vi "frontPanel.vi"(8 "error in (no error)":errorcluster, 10 "ScriptEvent":refnum<class "ScriptEvent.lvclass">, 11 "ActionPanel in":refnum<class "SingleToneRampAction.lvclass">) -> (0 "error out":errorcluster, 2 "ScriptEvent out":refnum<class "ScriptEvent.lvclass">, 3 "SingleToneRampAction out":refnum<class "SingleToneRampAction.lvclass">)   [LabVIEW 2011, in "Views.lvlib" / "ScriptEditor.lvlib" / "SingleToneRampAction.lvclass"]
uses:
  SingleToneRampAction.lvclass
  Tools/Scripting/ScriptingEvent/ScriptEvent.lvclass
  SingleToneRampAction.lvclass/SingleToneRampAction.ctl
  Tools/Scripting/ScriptingEvent/ScriptEvents/SingleTone/SingleToneRamp/SingleToneRamp.lvclass
  ActionPanel.lvclass
  Tools/Scripting/ScriptingEvent/ScriptEvents/SingleTone/SingleTone.lvclass
panel:
  in  "Stop Phase (Degrees)":dbl format="%#.6g"
  in  "Stop Frequency (kHz)":dbl format="%#.6g"
  in  "Stop Amplitude (Vpp)":string
  in  "Ramp Time":dbl format="%.6g"
  in  "Start Phase (Degrees)":dbl format="%#.6g"
  in  "Start Frequency (kHz)":dbl format="%#.6g"
  in  "Time":dbl format="%.6g"
  in  "Start Amplitude (Vpp)":string
  in  "Dt":dbl format="%.6g"
  out "editing":bool
  out "ready?":bool
  in  "close":bool
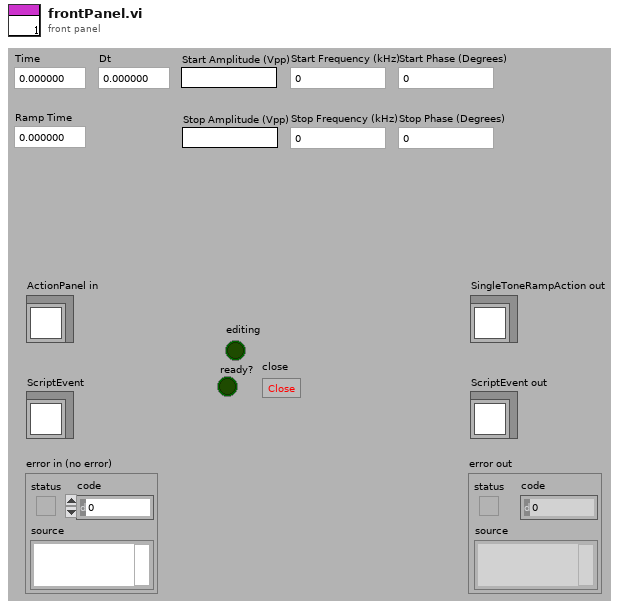
[diagram p1: front panel]
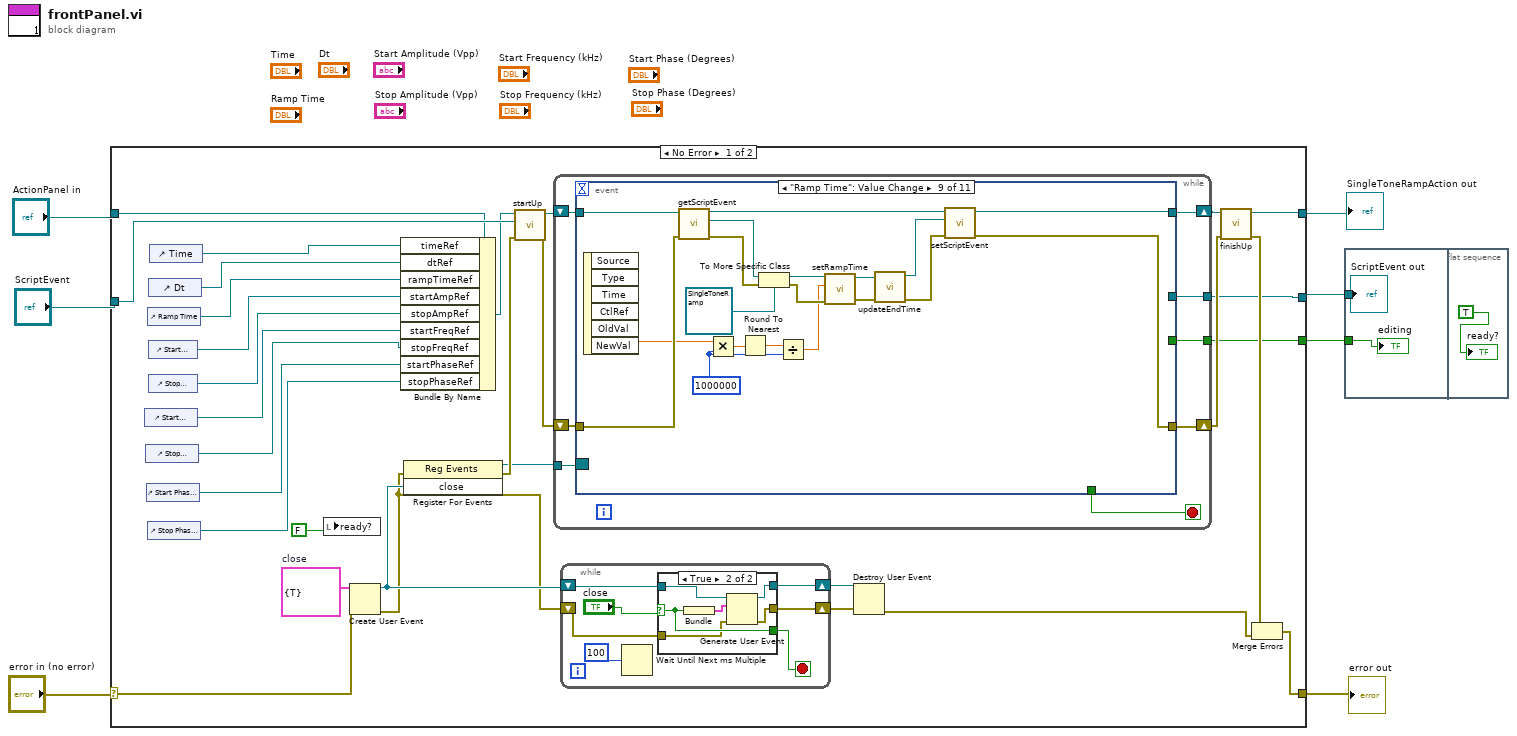
[diagram p0: block diagram]
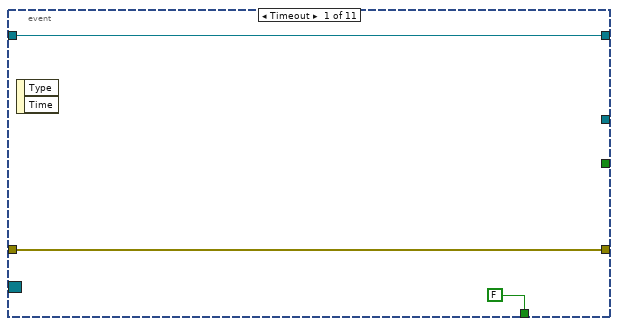
[diagram p3: hidden frame]
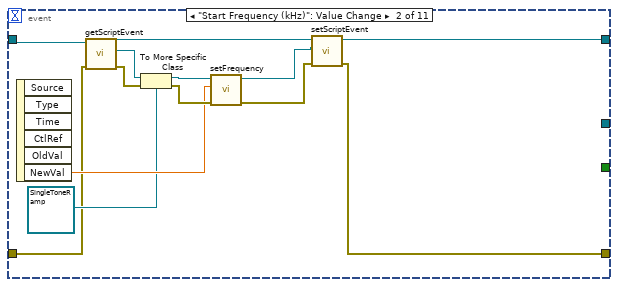
[diagram p4: hidden frame]
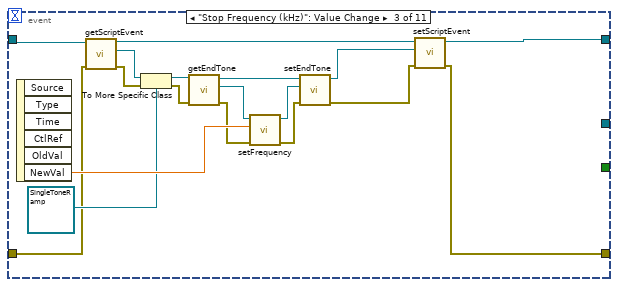
[diagram p5: hidden frame]
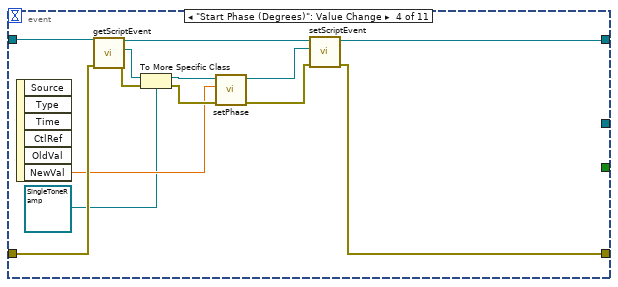
[diagram p6: hidden frame]
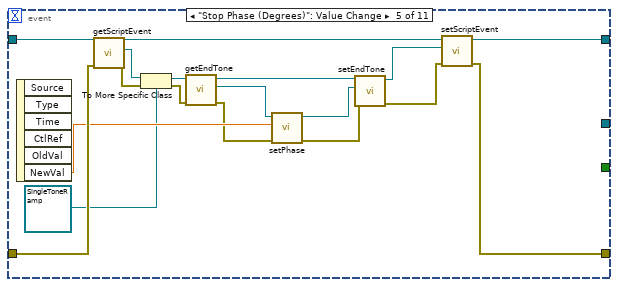
[diagram p7: hidden frame]
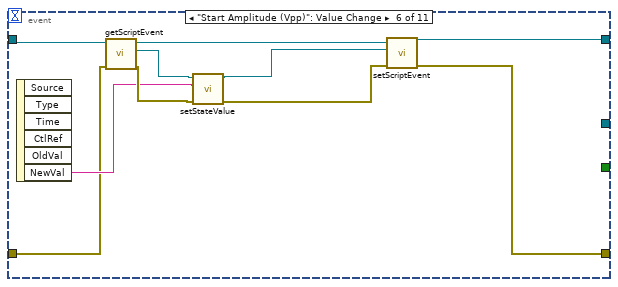
[diagram p8: hidden frame]
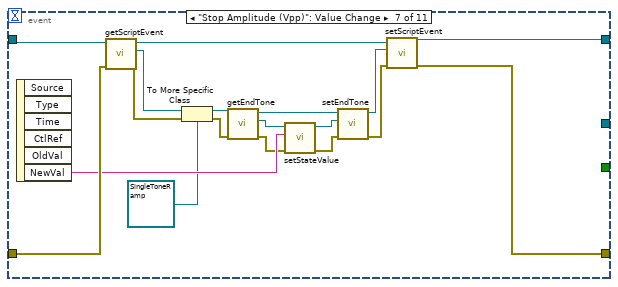
[diagram p9: hidden frame]
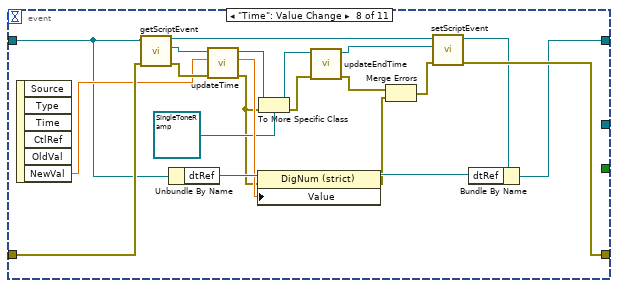
[diagram p10: hidden frame]
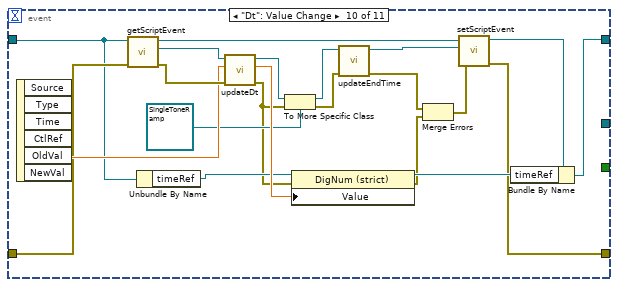
[diagram p11: hidden frame]
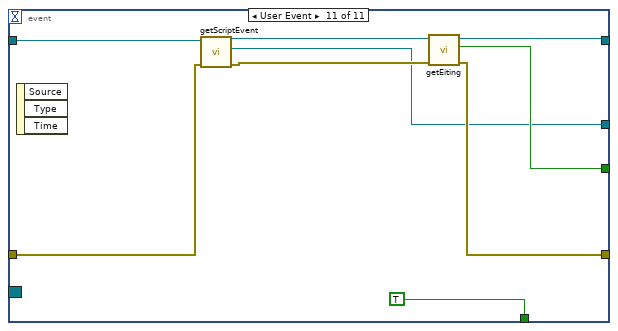
[diagram p12: hidden frame]
diagram:
  n1 = case shown="No Error" "error in (no error)" {
    selector: "error in (no error)" -> [w26 w226]
    tunnel: [w28 w226] -> w6
    tunnel: "ActionPanel in" -> [w9 w228]
    tunnel: [w38 w228] -> w1
    tunnel: "ScriptEvent" -> [w33 w227]
    tunnel: [w21 w227] -> w7
    tunnel: [w20 _] -> w2
    frame No Error {
      w27 = cluster{"close":bool} {"close"=TRUE}  # close
      n2 = control-ref of="Start Frequency (kHz)"() -> (w13:refnum<vi>)
      n3 = control-ref of="Stop Frequency (kHz)"() -> (w12:refnum<vi>)
      n4 = control-ref of="Start Phase (Degrees)"() -> (w11:refnum<vi>)
      n5 = control-ref of="Ramp Time"() -> (w16:refnum<vi>)
      n6 = control-ref of="Stop Phase (Degrees)"() -> (w10:refnum<vi>)
      n7 = control-ref of="Dt"() -> (w18:refnum<vi>)
      n8 = control-ref of="Start Amplitude (Vpp)"() -> (w15:refnum<vi>)
      n9 = control-ref of="Stop Amplitude (Vpp)"() -> (w14:refnum<vi>)
      n10 = control-ref of="Time"() -> (w19:refnum<vi>)
      n11 = local write "ready?"(FALSE) -> ()
      n12 = Create User Event(user event datatype=w27, error in=w26) -> (user event=w25:refnum<user-event>, error out=w24:errorcluster)
      n13 = Bundle By Name(cluster=w9, "timeRef"=w19, "dtRef"=w18, "rampTimeRef"=w16, "startAmpRef"=w15, "stopAmpRef"=w14, "startFreqRef"=w13, "stopFreqRef"=w12, "startPhaseRef"=w11, "stopPhaseRef"=w10) -> (w8:refnum<class "SingleToneRampAction.lvclass">)
      n14 = register-events(error in=w24, w25) -> (reference out=w22:refnum<event-registration>, error out=w23:errorcluster)  [unwired: 1 in]
      n15 = call-dynamic "startUp.vi"("error in (no error)"=w23, "ScriptEvent"=w33, "SingleToneRampAction in"=w8) -> ("error out"=w35:errorcluster, "SingleToneRampAction out"=w36:refnum<class "SingleToneRampAction.lvclass">)  [unwired: 7 in]
      n16 = while {
        shift-right: [w62] -> w37
        shift-left: w36 -> [w61]
        shift-right: [w59] -> w34
        shift-left: w35 -> [w60]
        tunnel: w22 -> [w57]
        tunnel: [w56] -> w21
        tunnel: [w55] -> w20
        stop <- w58 stop-if-true
        n17 = event shown="[8] \"Ramp Time\": Value Change" {
          selector: w57 -> [_ _ _ _ _ _ _ _ _ _ _]
          dyn-events: _ -> [_ _ _ _ _ _ _ _ _ _ _]
          timeout: _ -> [_ _ _ _ _ _ _ _ _ _ _]
          tunnel: [w64 w72 w92 w103 w121 w129 w152 w168 w182 w206 w222] -> w62
          tunnel: w61 -> [w64 w74 w94 w109 w127 w128 w151 w169 w192 w208 w223]
          tunnel: w60 -> [w63 w71 w91 w106 w124 w132 w154 w172 w194 w209 w220]
          tunnel: [w63 w66 w88 w104 w122 w131 w153 w170 w193 w211 w221] -> w59
          tunnel: [FALSE _ _ _ _ _ _ _ _ _ TRUE] -> w58
          tunnel: [_ _ _ _ _ _ _ _ _ _ w217] -> w56
          tunnel: [_ _ _ _ _ _ _ _ _ _ w219] -> w55
          event Timeout {
            n18 = event-data() -> ()  [unwired: 1 in, 2 out]
          }
          event "Start Frequency (kHz)": Value Change {
            n19 = event-data() -> ("NewVal"=w76:dbl)  [unwired: 1 in, 5 out]
            n20 = call "getScriptEvent.vi"("error in (no error)"=w71, "ActionPanel.lvclass in"=w74) -> ("error out"=w70:errorcluster, "ScriptEvent.lvclass"=w69:refnum<class "ScriptEvent.lvclass">, "ActionPanel.lvclass out"=w73:refnum<class "SingleToneRampAction.lvclass">)  [unwired: 7 in]
            n21 = To More Specific Class(target class=refnum<class "SingleToneRamp.lvclass"> refnum ("Tools.lvlib:Scripting.lvlib:SingleToneRamp.lvclass"), reference=w69, error in=w70) -> (specific class reference=w78:refnum<class "SingleToneRamp.lvclass">, error out=w77:errorcluster)
            n22 = call "setFrequency.vi"("error in (no error)"=w77, "frequency"=w76, "SingleTone.lvclass in"=w78) -> ("error out"=w67:errorcluster, "SingleTone.lvclass out"=w68:refnum<class "SingleToneRamp.lvclass">)  [unwired: 7 in]
            n23 = call "setScriptEvent.vi"("error in (no error)"=w67, "ScriptEvent.lvclass"=w68, "ActionPanel.lvclass in"=w73) -> ("error out"=w66:errorcluster, "ActionPanel.lvclass out"=w72:refnum<class "SingleToneRampAction.lvclass">)  [unwired: 7 in]
          }
          event "Stop Frequency (kHz)": Value Change {
            n24 = event-data() -> ("NewVal"=w96:dbl)  [unwired: 1 in, 5 out]
            n25 = call "getScriptEvent.vi"("error in (no error)"=w91, "ActionPanel.lvclass in"=w94) -> ("error out"=w90:errorcluster, "ScriptEvent.lvclass"=w89:refnum<class "ScriptEvent.lvclass">, "ActionPanel.lvclass out"=w93:refnum<class "SingleToneRampAction.lvclass">)  [unwired: 7 in]
            n26 = To More Specific Class(target class=refnum<class "SingleToneRamp.lvclass"> refnum ("Tools.lvlib:Scripting.lvlib:SingleToneRamp.lvclass"), reference=w89, error in=w90) -> (specific class reference=w87:refnum<class "SingleToneRamp.lvclass">, error out=w86:errorcluster)
            n27 = call "getEndTone.vi"("error in (no error)"=w86, "SingleToneRamp.lvclass in"=w87) -> ("error out"=w84:errorcluster, "endTone"=w85:refnum<class "SingleTone.lvclass">, "SingleToneRamp.lvclass out"=w83:refnum<class "SingleToneRamp.lvclass">)  [unwired: 7 in]
            n28 = call "setFrequency.vi"("error in (no error)"=w84, "frequency"=w96, "SingleTone.lvclass in"=w85) -> ("error out"=w82:errorcluster, "SingleTone.lvclass out"=w81:refnum<class "SingleTone.lvclass">)  [unwired: 7 in]
            n29 = call "setEndTone.vi"("error in (no error)"=w82, "EndTone"=w81, "SingleToneRamp.lvclass in"=w83) -> ("error out"=w79:errorcluster, "SingleToneRamp.lvclass out"=w80:refnum<class "SingleToneRamp.lvclass">)  [unwired: 7 in]
            n30 = call "setScriptEvent.vi"("error in (no error)"=w79, "ScriptEvent.lvclass"=w80, "ActionPanel.lvclass in"=w93) -> ("error out"=w88:errorcluster, "ActionPanel.lvclass out"=w92:refnum<class "SingleToneRampAction.lvclass">)  [unwired: 7 in]
          }
          event "Start Phase (Degrees)": Value Change {
            n31 = event-data() -> ("NewVal"=w98:dbl)  [unwired: 1 in, 5 out]
            n32 = call "getScriptEvent.vi"("error in (no error)"=w106, "ActionPanel.lvclass in"=w109) -> ("error out"=w107:errorcluster, "ScriptEvent.lvclass"=w108:refnum<class "ScriptEvent.lvclass">, "ActionPanel.lvclass out"=w105:refnum<class "SingleToneRampAction.lvclass">)  [unwired: 7 in]
            n33 = To More Specific Class(target class=refnum<class "SingleToneRamp.lvclass"> refnum ("Tools.lvlib:Scripting.lvlib:SingleToneRamp.lvclass"), reference=w108, error in=w107) -> (specific class reference=w102:refnum<class "SingleToneRamp.lvclass">, error out=w99:errorcluster)
            n34 = call "setPhase.vi"("error in (no error)"=w99, "phase"=w98, "SingleTone.lvclass in"=w102) -> ("error out"=w100:errorcluster, "SingleTone.lvclass out"=w101:refnum<class "SingleToneRamp.lvclass">)  [unwired: 7 in]
            n35 = call "setScriptEvent.vi"("error in (no error)"=w100, "ScriptEvent.lvclass"=w101, "ActionPanel.lvclass in"=w105) -> ("error out"=w104:errorcluster, "ActionPanel.lvclass out"=w103:refnum<class "SingleToneRampAction.lvclass">)  [unwired: 7 in]
          }
          event "Stop Phase (Degrees)": Value Change {
            n36 = event-data() -> ("NewVal"=w120:dbl)  [unwired: 1 in, 5 out]
            n37 = call "getScriptEvent.vi"("error in (no error)"=w124, "ActionPanel.lvclass in"=w127) -> ("error out"=w125:errorcluster, "ScriptEvent.lvclass"=w126:refnum<class "ScriptEvent.lvclass">, "ActionPanel.lvclass out"=w123:refnum<class "SingleToneRampAction.lvclass">)  [unwired: 7 in]
            n38 = To More Specific Class(target class=refnum<class "SingleToneRamp.lvclass"> refnum ("Tools.lvlib:Scripting.lvlib:SingleToneRamp.lvclass"), reference=w126, error in=w125) -> (specific class reference=w114:refnum<class "SingleToneRamp.lvclass">, error out=w113:errorcluster)
            n39 = call "getEndTone.vi"("error in (no error)"=w113, "SingleToneRamp.lvclass in"=w114) -> ("error out"=w112:errorcluster, "endTone"=w115:refnum<class "SingleTone.lvclass">, "SingleToneRamp.lvclass out"=w116:refnum<class "SingleToneRamp.lvclass">)  [unwired: 7 in]
            n40 = call "setPhase.vi"("error in (no error)"=w112, "phase"=w120, "SingleTone.lvclass in"=w115) -> ("error out"=w117:errorcluster, "SingleTone.lvclass out"=w118:refnum<class "SingleTone.lvclass">)  [unwired: 7 in]
            n41 = call "setEndTone.vi"("error in (no error)"=w117, "EndTone"=w118, "SingleToneRamp.lvclass in"=w116) -> ("error out"=w110:errorcluster, "SingleToneRamp.lvclass out"=w111:refnum<class "SingleToneRamp.lvclass">)  [unwired: 7 in]
            n42 = call "setScriptEvent.vi"("error in (no error)"=w110, "ScriptEvent.lvclass"=w111, "ActionPanel.lvclass in"=w123) -> ("error out"=w122:errorcluster, "ActionPanel.lvclass out"=w121:refnum<class "SingleToneRampAction.lvclass">)  [unwired: 7 in]
          }
          event "Start Amplitude (Vpp)": Value Change {
            n43 = event-data() -> ("NewVal"=w133:string)  [unwired: 1 in, 5 out]
            n44 = call "getScriptEvent.vi"("error in (no error)"=w132, "ActionPanel.lvclass in"=w128) -> ("error out"=w134:errorcluster, "ScriptEvent.lvclass"=w136:refnum<class "ScriptEvent.lvclass">, "ActionPanel.lvclass out"=w137:refnum<class "SingleToneRampAction.lvclass">)  [unwired: 7 in]
            n45 = call "setStateValue.vi"("error in (no error)"=w134, "stateValue"=w133, "ScriptEvent in"=w136) -> ("error out"=w130:errorcluster, "ScriptEvent out"=w135:refnum<class "ScriptEvent.lvclass">)  [unwired: 7 in]
            n46 = call "setScriptEvent.vi"("error in (no error)"=w130, "ScriptEvent.lvclass"=w135, "ActionPanel.lvclass in"=w137) -> ("error out"=w131:errorcluster, "ActionPanel.lvclass out"=w129:refnum<class "SingleToneRampAction.lvclass">)  [unwired: 7 in]
          }
          event "Stop Amplitude (Vpp)": Value Change {
            n47 = event-data() -> ("NewVal"=w147:string)  [unwired: 1 in, 5 out]
            n48 = call "getScriptEvent.vi"("error in (no error)"=w154, "ActionPanel.lvclass in"=w151) -> ("error out"=w144:errorcluster, "ScriptEvent.lvclass"=w146:refnum<class "ScriptEvent.lvclass">, "ActionPanel.lvclass out"=w155:refnum<class "SingleToneRampAction.lvclass">)  [unwired: 7 in]
            n49 = To More Specific Class(target class=refnum<class "SingleToneRamp.lvclass"> refnum ("Tools.lvlib:Scripting.lvlib:SingleToneRamp.lvclass"), reference=w146, error in=w144) -> (specific class reference=w150:refnum<class "SingleToneRamp.lvclass">, error out=w149:errorcluster)
            n50 = call "getEndTone.vi"("error in (no error)"=w149, "SingleToneRamp.lvclass in"=w150) -> ("error out"=w143:errorcluster, "endTone"=w148:refnum<class "SingleTone.lvclass">, "SingleToneRamp.lvclass out"=w142:refnum<class "SingleToneRamp.lvclass">)  [unwired: 7 in]
            n51 = call "setStateValue.vi"("error in (no error)"=w143, "stateValue"=w147, "ScriptEvent in"=w148) -> ("error out"=w140:errorcluster, "ScriptEvent out"=w141:refnum<class "SingleTone.lvclass">)  [unwired: 7 in]
            n52 = call "setEndTone.vi"("error in (no error)"=w140, "EndTone"=w141, "SingleToneRamp.lvclass in"=w142) -> ("error out"=w138:errorcluster, "SingleToneRamp.lvclass out"=w139:refnum<class "SingleToneRamp.lvclass">)  [unwired: 7 in]
            n53 = call "setScriptEvent.vi"("error in (no error)"=w138, "ScriptEvent.lvclass"=w139, "ActionPanel.lvclass in"=w155) -> ("error out"=w153:errorcluster, "ActionPanel.lvclass out"=w152:refnum<class "SingleToneRampAction.lvclass">)  [unwired: 7 in]
          }
          event "Time": Value Change {
            n54 = event-data() -> ("NewVal"=w171:dbl)  [unwired: 1 in, 5 out]
            n55 = call "getScriptEvent.vi"("error in (no error)"=w172, "ActionPanel.lvclass in"=w169) -> ("error out"=w174:errorcluster, "ScriptEvent.lvclass"=w175:refnum<class "ScriptEvent.lvclass">, "ActionPanel.lvclass out"=w176:refnum<class "SingleToneRampAction.lvclass">)  [unwired: 7 in]
            n56 = Unbundle By Name(w169) -> ("dtRef"=w166:refnum<vi>)
            n57 = call "updateTime.vi"("error in (no error)"=w174, "time"=w171, "ScriptEvent in"=w175) -> ("error out"=w161:errorcluster, "dt"=w165:dbl, "ScriptEvent out"=w162:refnum<class "ScriptEvent.lvclass">)  [unwired: 6 in]
            n58 = property class="DigNum (strict)"(reference=w166, error in=w161, "Value"=w165) -> (reference out=w173:refnum<vi>, error out=w157:errorcluster)
            n59 = To More Specific Class(target class=refnum<class "SingleToneRamp.lvclass"> refnum ("Tools.lvlib:Scripting.lvlib:SingleToneRamp.lvclass"), reference=w162, error in=w161) -> (specific class reference=w160:refnum<class "SingleToneRamp.lvclass">, error out=w164:errorcluster)
            n60 = call-dynamic "updateEndTime.vi"("error in (no error)"=w164, "SingleToneRamp in"=w160) -> ("error out"=w158:errorcluster, "SingleToneRamp out"=w159:refnum<class "SingleToneRamp.lvclass">)  [unwired: 8 in]
            n61 = Merge Errors(w158, w157) -> (w156:errorcluster)
            n62 = call "setScriptEvent.vi"("error in (no error)"=w156, "ScriptEvent.lvclass"=w159, "ActionPanel.lvclass in"=w176) -> ("error out"=w170:errorcluster, "ActionPanel.lvclass out"=w167:refnum<class "SingleToneRampAction.lvclass">)  [unwired: 7 in]
            n63 = Bundle By Name(cluster=w167, "dtRef"=w173) -> (w168:refnum<class "SingleToneRampAction.lvclass">)
          }
          event "Ramp Time": Value Change {
            w179 = 1000000
            n64 = event-data() -> ("NewVal"=w178:dbl)  [unwired: 1 in, 5 out]
            n65 = call "getScriptEvent.vi"("error in (no error)"=w194, "ActionPanel.lvclass in"=w192) -> ("error out"=w188:errorcluster, "ScriptEvent.lvclass"=w190:refnum<class "ScriptEvent.lvclass">, "ActionPanel.lvclass out"=w195:refnum<class "SingleToneRampAction.lvclass">)  [unwired: 7 in]
            n66 = Multiply(x=w178, y=w179) -> (x*y=w181:dbl)
            n67 = Round To Nearest(number=w181) -> (nearest integer value=w180:dbl)
            n68 = To More Specific Class(target class=refnum<class "SingleToneRamp.lvclass"> refnum ("Tools.lvlib:Scripting.lvlib:SingleToneRamp.lvclass"), reference=w190, error in=w188) -> (specific class reference=w187:refnum<class "SingleToneRamp.lvclass">, error out=w186:errorcluster)
            n69 = Divide(x=w180, y=w179) -> (x/y=w177:dbl)
            n70 = call "setRampTime.vi"("error in (no error)"=w186, "rampTime"=w177, "SingleToneRamp.lvclass in"=w187) -> ("error out"=w184:errorcluster, "SingleToneRamp.lvclass out"=w185:refnum<class "SingleToneRamp.lvclass">)  [unwired: 7 in]
            n71 = call-dynamic "updateEndTime.vi"("error in (no error)"=w184, "SingleToneRamp in"=w185) -> ("error out"=w183:errorcluster, "SingleToneRamp out"=w191:refnum<class "SingleToneRamp.lvclass">)  [unwired: 8 in]
            n72 = call "setScriptEvent.vi"("error in (no error)"=w183, "ScriptEvent.lvclass"=w191, "ActionPanel.lvclass in"=w195) -> ("error out"=w193:errorcluster, "ActionPanel.lvclass out"=w182:refnum<class "SingleToneRampAction.lvclass">)  [unwired: 7 in]
          }
          event "Dt": Value Change {
            n73 = event-data() -> ("NewVal"=w210:dbl)  [unwired: 1 in, 5 out]
            n74 = call "getScriptEvent.vi"("error in (no error)"=w209, "ActionPanel.lvclass in"=w208) -> ("error out"=w213:errorcluster, "ScriptEvent.lvclass"=w214:refnum<class "ScriptEvent.lvclass">, "ActionPanel.lvclass out"=w216:refnum<class "SingleToneRampAction.lvclass">)  [unwired: 7 in]
            n75 = Unbundle By Name(w208) -> ("timeRef"=w205:refnum<vi>)
            n76 = call "updateDt.vi"("error in (no error)"=w213, "dt"=w210, "ScriptEvent in"=w214) -> ("error out"=w200:errorcluster, "time"=w212:dbl, "ScriptEvent out"=w203:refnum<class "ScriptEvent.lvclass">)  [unwired: 6 in]
            n77 = To More Specific Class(target class=refnum<class "SingleToneRamp.lvclass"> refnum ("Tools.lvlib:Scripting.lvlib:SingleToneRamp.lvclass"), reference=w203, error in=w200) -> (specific class reference=w201:refnum<class "SingleToneRamp.lvclass">, error out=w199:errorcluster)
            n78 = property class="DigNum (strict)"(reference=w205, error in=w200, "Value"=w212) -> (reference out=w215:refnum<vi>, error out=w197:errorcluster)
            n79 = call-dynamic "updateEndTime.vi"("error in (no error)"=w199, "SingleToneRamp in"=w201) -> ("error out"=w198:errorcluster, "SingleToneRamp out"=w204:refnum<class "SingleToneRamp.lvclass">)  [unwired: 8 in]
            n80 = Merge Errors(w198, w197) -> (w196:errorcluster)
            n81 = call "setScriptEvent.vi"("error in (no error)"=w196, "ScriptEvent.lvclass"=w204, "ActionPanel.lvclass in"=w216) -> ("error out"=w211:errorcluster, "ActionPanel.lvclass out"=w207:refnum<class "SingleToneRampAction.lvclass">)  [unwired: 7 in]
            n82 = Bundle By Name(cluster=w207, "timeRef"=w215) -> (w206:refnum<class "SingleToneRampAction.lvclass">)
          }
          event User Event {
            n83 = event-data() -> ()  [unwired: 1 in, 3 out]
            n84 = call "getScriptEvent.vi"("error in (no error)"=w220, "ActionPanel.lvclass in"=w223) -> ("error out"=w224:errorcluster, "ScriptEvent.lvclass"=w217:refnum<class "ScriptEvent.lvclass">, "ActionPanel.lvclass out"=w225:refnum<class "SingleToneRampAction.lvclass">)  [unwired: 7 in]
            n85 = call "getEiting.vi"("error in (no error)"=w224, "ActionPanel.lvclass in"=w225) -> ("error out"=w221:errorcluster, "editing?"=w219:bool, "ActionPanel.lvclass out"=w222:refnum<class "SingleToneRampAction.lvclass">)  [unwired: 7 in]
          }
        }
      }
      n86 = while {
        shift-right: [w42] -> w31
        shift-left: w24 -> [w41]
        shift-right: [w43] -> w32
        shift-left: w25 -> [w45]
        stop <- w44 stop-if-true
        n87 = Wait Until Next ms Multiple(millisecond multiple=100) -> ()  [unwired: 1 out]
        n88 = case shown="True" "close" {
          selector: "close" -> [w48 w52]
          tunnel: w45 -> [w47 w54]
          tunnel: [w48 w52] -> w44
          tunnel: [w47 w51] -> w43
          tunnel: [w46 w50] -> w42
          tunnel: w41 -> [w46 w49]
          frame False {
          }
          frame True {
            n89 = Bundle(w52) -> (w53:cluster{bool})  [unwired: 1 in]
            n90 = Generate User Event(user event=w54, event data cluster=w53, error in=w49) -> (user event out=w51:refnum<user-event>, error out=w50:errorcluster)
          }
        }
      }
      n91 = Destroy User Event(user event=w32, error in=w31) -> (error out=w29:errorcluster)
      n92 = call-dynamic "finishUp.vi"("error in (no error)"=w34, "SingleToneRampAction in"=w37) -> ("error out"=w30:errorcluster, "SingleToneRampAction out"=w38:refnum<class "SingleToneRampAction.lvclass">)  [unwired: 8 in]
      n93 = Merge Errors(w30, w29) -> (w28:errorcluster)
    }
    frame Error {
    }
  }
  "error out" <- w6
  "SingleToneRampAction out" <- w1
  n94 = flat-sequence {
    tunnel: w7 -> [w230]
    tunnel: w2 -> [w229]
    frame #0 {
      "ScriptEvent out" <- w230
      "editing" <- w229
    }
    frame #1 {
      "ready?" <- TRUE
    }
  }
